vi "系统设置.vi"() -> ()   [LabVIEW 2016]
uses:
  <vilib>/Utility/miscctls.llb/LVPointTypeDef.ctl
  <vilib>/ptbypt/NI_PtbyPt.lvlib
  <vilib>/Utility/config.llb/NI_LVConfig.lvlib
  PLC/PLC.lvlib
panel:
  out "二级权限":bool
  in  "定时重启配置":bool
  in  "模块启用配置":bool
  in  "短信报警设置":bool
  in  "首页显示设置":bool
  in  "跨度核查":bool
  in  "空白核查":bool
  out "选项卡控件":enum32{"自由设定", "国标协议", "流量设定"}(tab)
  in  "24H周期设置":bool[](xcontrol)
  in  "运行间隔":i16=4 min=1 max=24
  in  "流量阈值":dbl=4.0 min=1.0 max=24.0
  in  "时间阈值":u16=4 min=1 max=24
  in  "周期设置":enum16{"自由设定", "国标协议", "流量设定"}(ring)
  out "一级权限":bool
  in  "质控启动日期":string(combo)="关闭"
  in  "跨度核查时间":u16(ring)=6 items=["00H", "01H", "02H", "03H", "04H", "05H", "06H", "07H", "08H", "09H", "10H", "11H", "12H", "13H", "14H", "15H", "16H", "17H", "18H", "19H", "20H", "21H", "22H", "23H", "关闭"]
  in  "空白核查时间":u16(ring)=2 items=["00H", "01H", "02H", "03H", "04H", "05H", "06H", "07H", "08H", "09H", "10H", "11H", "12H", "13H", "14H", "15H", "16H", "17H", "18H", "19H", "20H", "21H", "22H", "23H", "关闭"]
  in  "CODCr":bool
  in  "总磷总氮":bool
  in  "氨氮":bool
  in  "CODmn":bool
  in  "多参数":bool
  in  "输入密码":u32
  in  "布尔":bool
  in  "副屏显示设置":bool
  in  "开机启动":bool caption="氨氮禁用"
  in  "运行模式":enum16{"维护模式", "常规模式", "应急模式", "质控模式"}(ring)
  # "注：周期设置分为自由设定和国标协议两种。\n1：选择自由设定情况下：运行间隔将不可选用并变灰色，周期设置可自由手动勾选\n2：选择国标协议情况下：周期时间将由运行间隔选择的时间决定，下方周期设置被禁用并无法手动勾选。\n3：选择流量设定情况下：瞬时流量连续超过流量阈值到达时间阈值设定值，仪器将自动开启测量。"
  # "自动运行启动参数"
  # "质控频次："
  # "零点核查时间："
  # "跨度核查时间："
  # "启动周期设置"
  # "m3/S"
  # "秒"
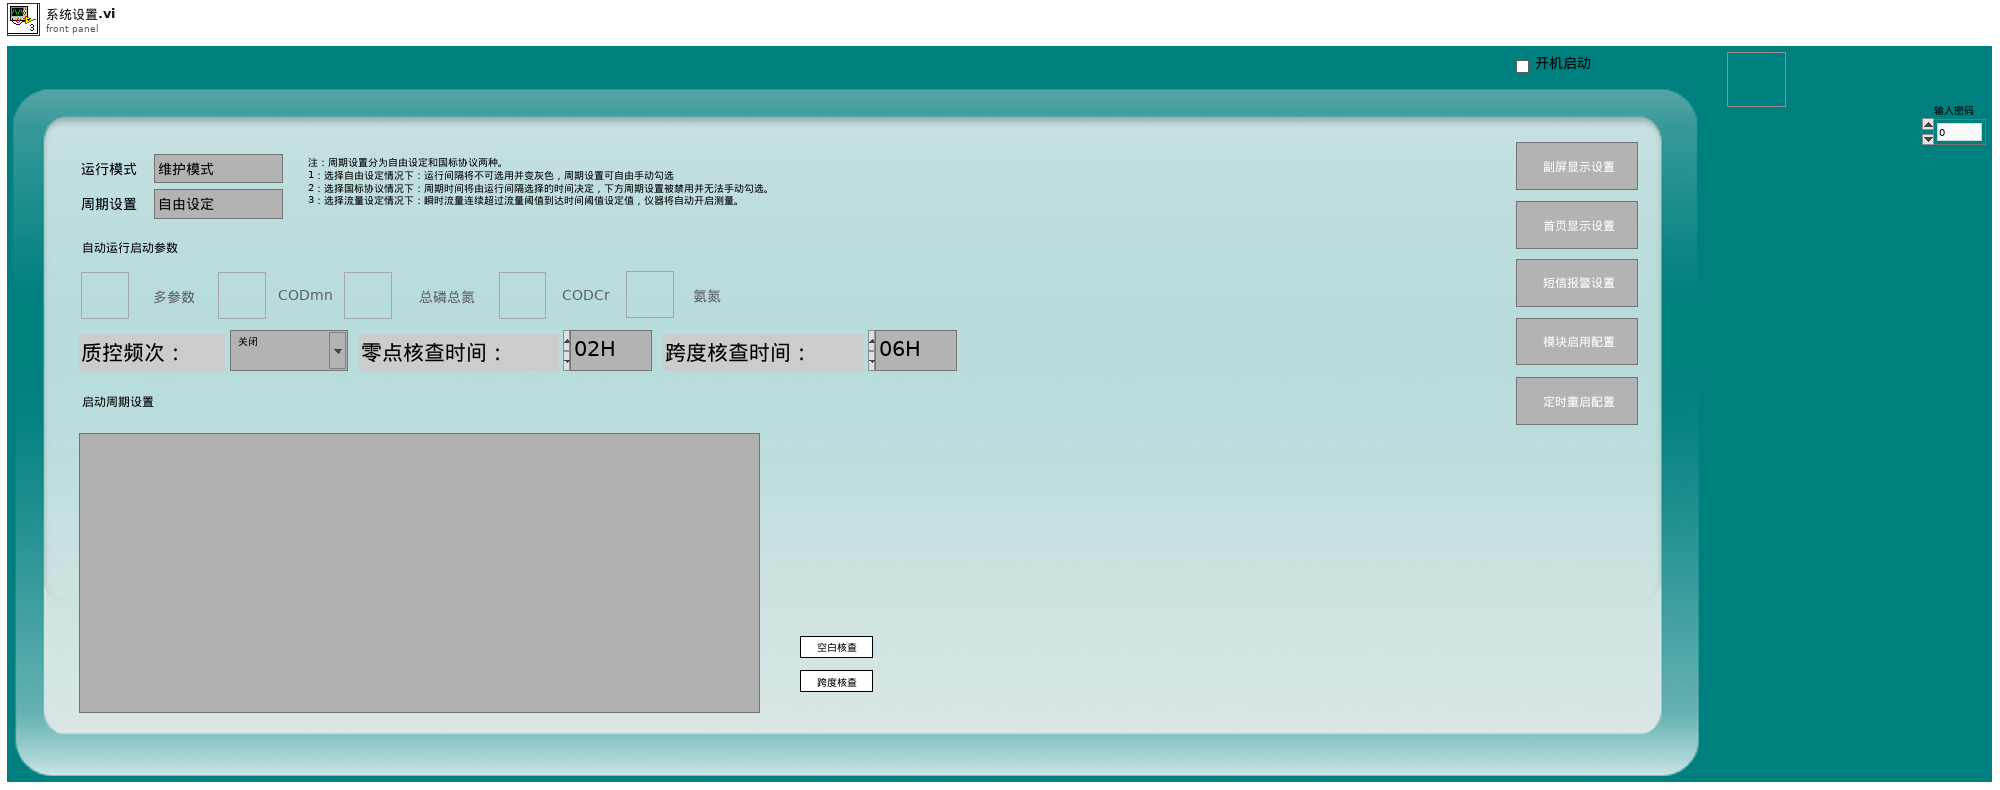
[diagram p1: front panel]
types:
  T1 = typedef "LVPointTypeDef.ctl" = cluster{"Horizontal":i16, "Vertical":i16}
  T2 = enum8{"Enabled", "Disabled", "Disabled and Grayed Out"}
  T3 = cluster{"频次":enum16{"关闭", "每天", "星期一", "星期二", "星期三", "星期四", "星期五", "星期六", "星期日"}, "时":u16, "分":u16}
  T4 = typedef "LVDateTimeRec.ctl" = cluster{"秒数的小数部分":dbl, "秒":i32, "分":i32, "时":i32, "日":i32, "月":i32, "年":i32, "天数（周）":i32, "天数（年）":i32, "DST":i32}
  T5 = enum16{"关闭", "每天", "星期一", "星期二", "星期三", "星期四", "星期五", "星期六", "星期日"}
  T6 = enum32{"Bad", "Idle", "Run top level", "Running"}
  T7 = typedef "NI_LVConfig.lvlib/Config Data RefNum.ctl" = refnum<k1>
  T8 = cluster{"运行模式":enum16{"维护模式", "常规模式", "应急模式", "质控模式"}}
  T9 = cluster{"测量模式":enum16{"水样测量", "标样核查", "零点核查", "跨度核查", "空白测试", "加标回收", "平行样", "校零", "校标"}}
  T10 = enum16{"启动测量", "标样核查", "零点核查", "跨度核查", "空白测试", "平行样测试", "加标回收", "空白校准", "标样校准", "初始化（清洗）", "停止测试", "仪器重启", "校时", "模式设置", "测量间隔设置"}
  T11 = cluster{"测试模式":enum16{"正常测试", "集成干预"}, "参数启用":cluster{"氨氮":bool, "总磷总氮":bool, "CODMn":bool, "CODcr":bool, "多参数":bool}}
  T12 = cluster{"运行模式":enum16{"维护模式", "常规模式", "应急模式", "质控模式"}, "质控频次":enum16{"关闭", "每天", "星期一", "星期二", "星期三", "星期四", "星期五", "星期六", "星期日"}, "空白核查时间":u16, "跨度核查时间":u16, "24H周期设置":bool[]}
  T13 = enum32{"Invalid", "Standard", "Closed", "Hidden", "Minimized", "Maximized"}
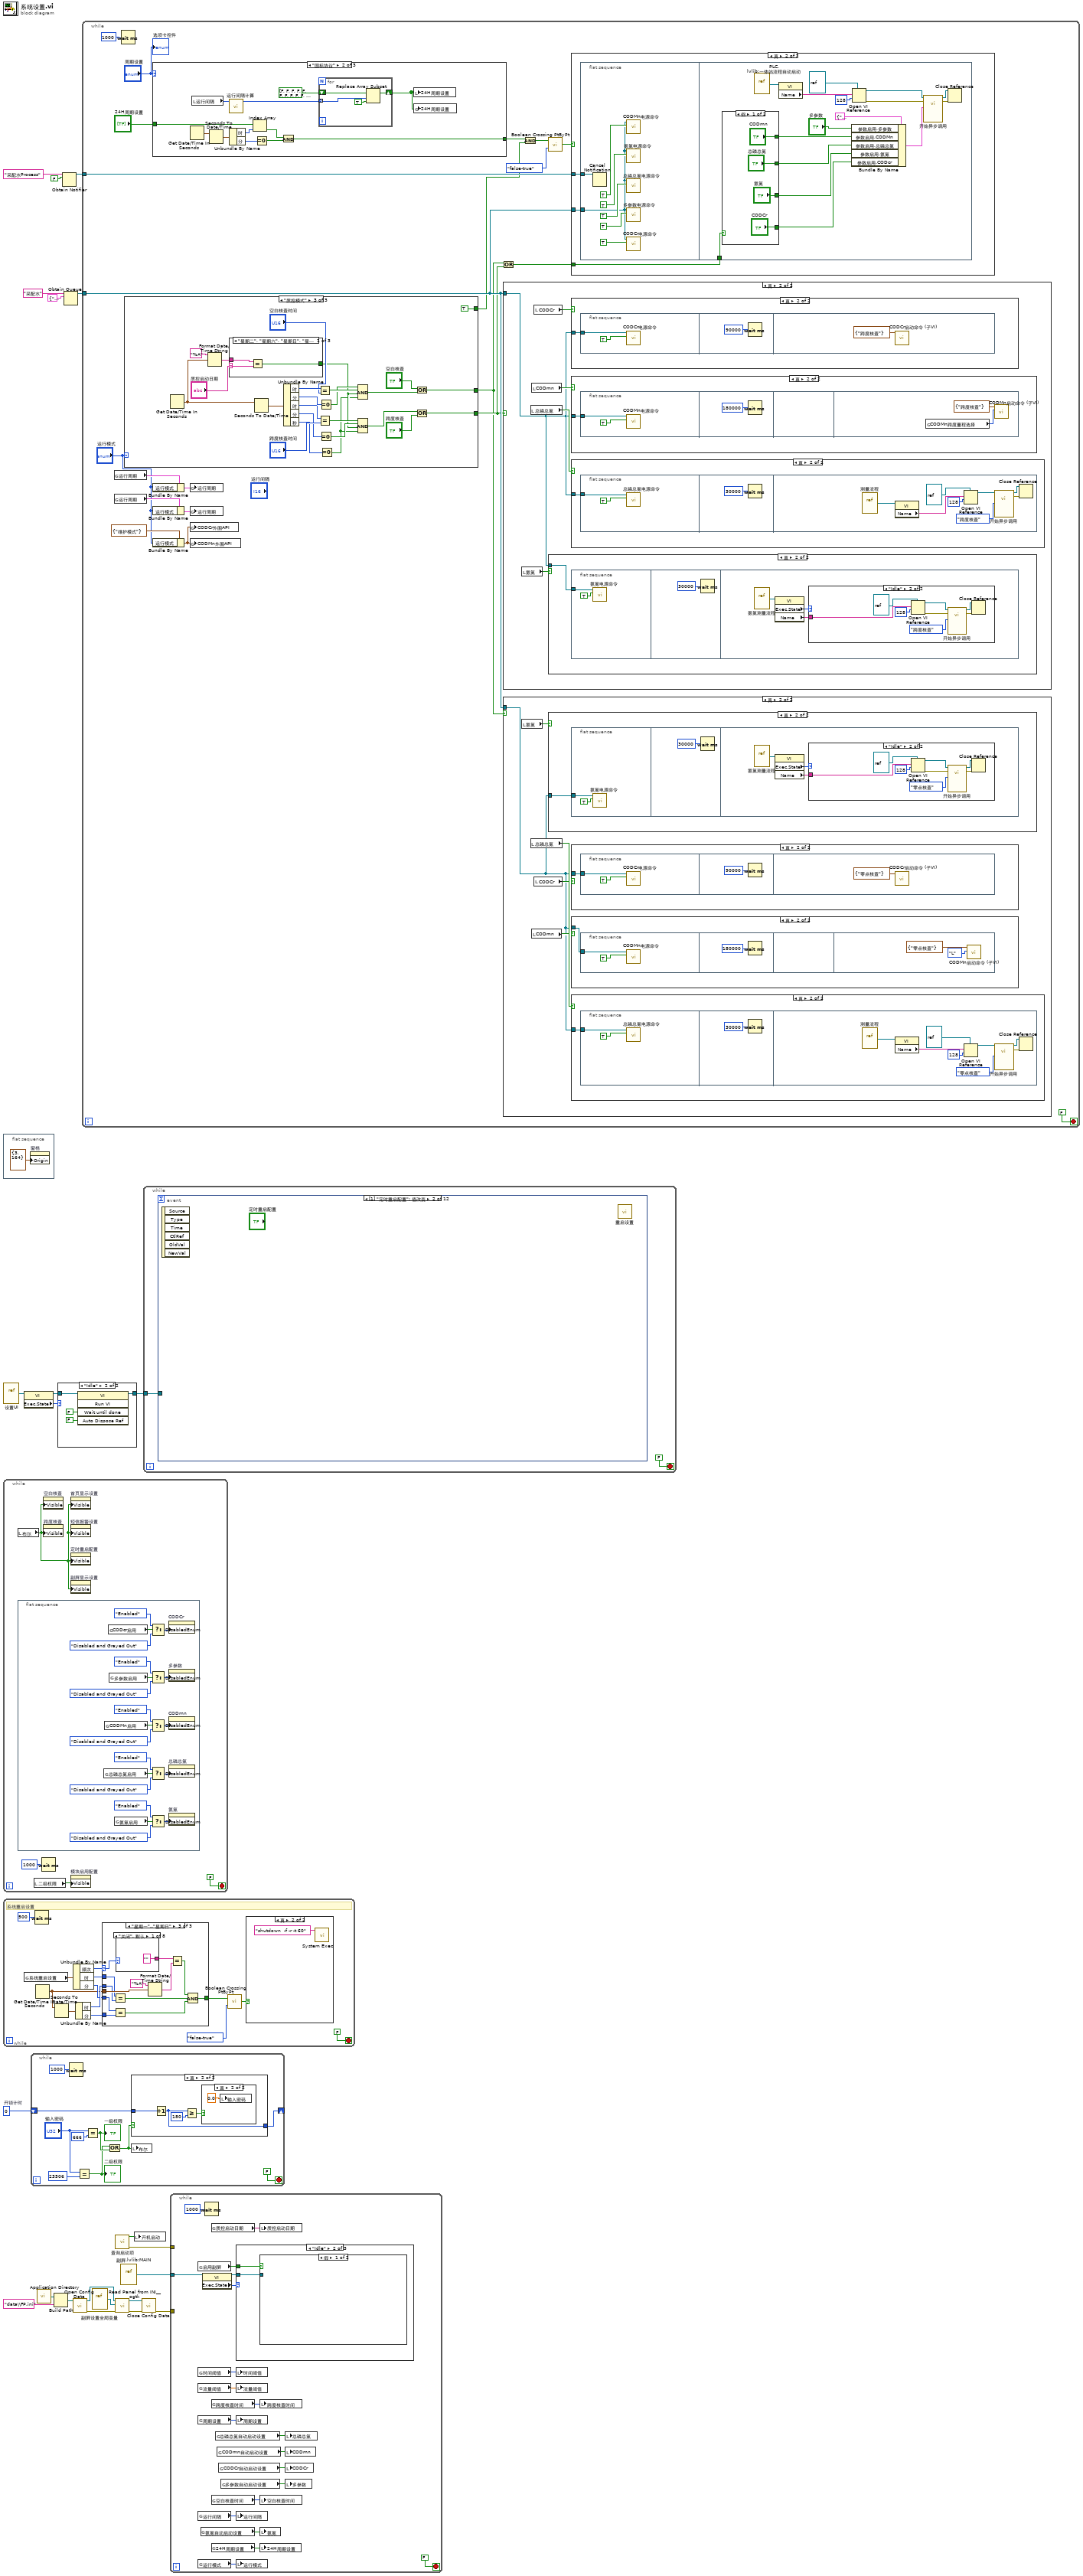
[diagram p0: block diagram]
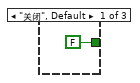
[diagram p3: hidden frame]
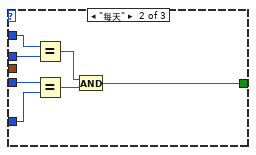
[diagram p4: hidden frame]
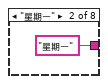
[diagram p5: hidden frame]
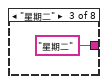
[diagram p6: hidden frame]
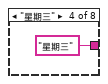
[diagram p7: hidden frame]
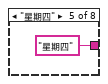
[diagram p8: hidden frame]
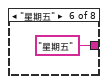
[diagram p9: hidden frame]
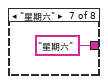
[diagram p10: hidden frame]
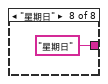
[diagram p11: hidden frame]
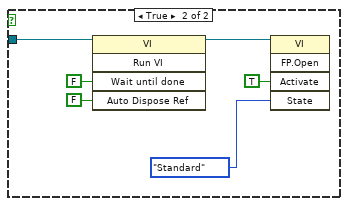
[diagram p16: hidden frame]
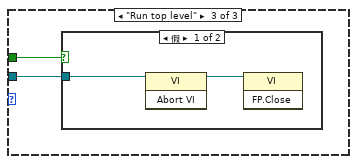
[diagram p17: hidden frame]
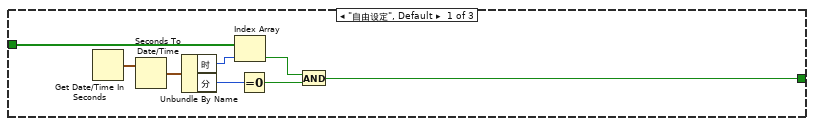
[diagram p19: hidden frame]
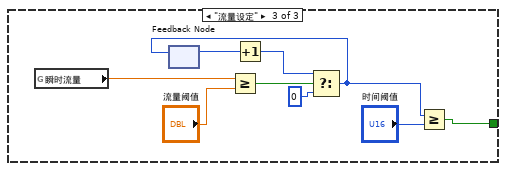
[diagram p20: hidden frame]
diagram:
  w19 = u32 0  # 开锁计时
  n1 = flat-sequence {
    frame #0 {
      n2 = property on="窗格" class="Pane"("Origin"=T1 {"Horizontal"=3, "Vertical"=164} ("原点")) -> ()  [unwired: 2 in, 2 out]
    }
  }
  n3 = vi-ref "设置UI.vi"() -> (w14:refnum<vi>)
  n4 = while {
    stop <- FALSE stop-if-true
    n5 = local read "布尔"() -> (w25:bool)
    n6 = flat-sequence {
      frame #0 {
        n7 = global read "系统设置全局变量.vi" "总磷总氮启用"() -> (w36:bool)
        n8 = global read "系统设置全局变量.vi" "CODMn启用"() -> (w34:bool)
        n9 = global read "系统设置全局变量.vi" "CODcr启用"() -> (w35:bool)
        n10 = global read "系统设置全局变量.vi" "多参数启用"() -> (w33:bool)
        n11 = global read "系统设置全局变量.vi" "氨氮启用"() -> (w29:bool)
        n12 = Select(t=T2."Enabled" ("禁用"), s=w35, f=T2."Disabled and Grayed Out" ("禁用")) -> (s? t:f=w48:T2)
        n13 = Select(t=T2."Enabled" ("禁用"), s=w33, f=T2."Disabled and Grayed Out" ("禁用")) -> (s? t:f=w32:T2)
        n14 = Select(t=T2."Enabled" ("禁用"), s=w34, f=T2."Disabled and Grayed Out" ("禁用")) -> (s? t:f=w38:T2)
        n15 = Select(t=T2."Enabled" ("禁用"), s=w36, f=T2."Disabled and Grayed Out" ("禁用")) -> (s? t:f=w31:T2)
        n16 = Select(t=T2."Enabled" ("禁用"), s=w29, f=T2."Disabled and Grayed Out" ("禁用")) -> (s? t:f=w37:T2)
        n17 = property on="CODCr" class="Bool (严格)"("DisabledEnum"=w48) -> ()  [unwired: 2 in, 2 out]
        n18 = property on="多参数" class="Bool (严格)"("DisabledEnum"=w32) -> ()  [unwired: 2 in, 2 out]
        n19 = property on="CODmn" class="Bool (严格)"("DisabledEnum"=w38) -> ()  [unwired: 2 in, 2 out]
        n20 = property on="总磷总氮" class="Bool (严格)"("DisabledEnum"=w31) -> ()  [unwired: 2 in, 2 out]
        n21 = property on="氨氮" class="Bool (严格)"("DisabledEnum"=w37) -> ()  [unwired: 2 in, 2 out]
      }
    }
    n22 = local read "二级权限"() -> (w26:bool)
    n23 = Wait (ms)(milliseconds to wait=u32 1000 ("等待时间（毫秒）")) -> ()  [unwired: 1 out]
    n24 = property on="空白核查" class="Bool"("Visible"=w25) -> ()  [unwired: 2 in, 2 out]
    n25 = property on="跨度核查" class="Bool"("Visible"=w25) -> ()  [unwired: 2 in, 2 out]
    n26 = property on="首页显示设置" class="Bool"("Visible"=w25) -> ()  [unwired: 2 in, 2 out]
    n27 = property on="短信报警设置" class="Bool"("Visible"=w25) -> ()  [unwired: 2 in, 2 out]
    n28 = property on="定时重启配置" class="Bool"("Visible"=w25) -> ()  [unwired: 2 in, 2 out]
    n29 = property on="副屏显示设置" class="Bool"("Visible"=w25) -> ()  [unwired: 2 in, 2 out]
    n30 = property on="模块启用配置" class="Bool"("Visible"=w26) -> ()  [unwired: 2 in, 2 out]
  }
  n31 = while {
    stop <- FALSE stop-if-true
    # "系统重启设置"
    n32 = global read "系统设置全局变量.vi" "系统重启设置"() -> (w61:T3)
    n33 = Wait (ms)(milliseconds to wait=u32 500 ("等待时间（毫秒）")) -> ()  [unwired: 1 out]
    n34 = Get Date/Time In Seconds() -> (seconds since 1Jan1904=w52:timestamp)
    n35 = Seconds To Date/Time(time stamp (now)=w52) -> (date time rec=w59:T4)  [unwired: 1 in]
    n36 = Unbundle By Name(w61) -> ("频次"=w60:T5, "时"=w56:u16, "分"=w55:u16)
    n37 = Unbundle By Name(w59) -> ("时"=w58:i32, "分"=w57:i32)
    n38 = case shown="\"星期一\"..\"星期日\"" w60 {
      selector: w60 -> [_ _ w81]
      tunnel: [FALSE w64 w71] -> w51
      tunnel: w58 -> [_ w70 w75]
      tunnel: w57 -> [_ w67 w73]
      tunnel: w56 -> [_ w69 w76]
      tunnel: w55 -> [_ w68 w74]
      tunnel: w52 -> [_ _ w82]
      frame "关闭", Default {
      }
      frame "每天" {
        n39 = Equal?(x=w69, y=w70) -> (x = y?=w65:bool)
        n40 = Equal?(x=w68, y=w67) -> (x = y?=w66:bool)
        n41 = And(x=w65, y=w66) -> (x .and. y?=w64:bool)
      }
      frame "星期一".."星期日" {
        n42 = Equal?(x=w76, y=w75) -> (x = y?=w77:bool)
        n43 = Equal?(x=w74, y=w73) -> (x = y?=w78:bool)
        n44 = case shown="\"关闭\", 默认" w81 {
          tunnel: ["" ("时间格式字符串(%c)") "星期一" ("时间格式字符串(%c)") "星期二" ("时间格式字符串(%c)") "星期三" ("时间格式字符串(%c)") "星期四" ("时间格式字符串(%c)") "星期五" ("时间格式字符串(%c)") "星期六" ("时间格式字符串(%c)") "星期日" ("时间格式字符串(%c)")] -> w79
          frame "关闭", Default {
          }
          frame "星期一" {
          }
          frame "星期二" {
          }
          frame "星期三" {
          }
          frame "星期四" {
          }
          frame "星期五" {
          }
          frame "星期六" {
          }
          frame "星期日" {
          }
        }
        n45 = Format Date/Time String(time format string (%c)="%A" ("时间格式字符串(%c)"), seconds (now)=w82) -> (date/time string=w80:string)  [unwired: 1 in]
        n46 = Equal?(x=w79, y=w80) -> (x = y?=w72:bool)
        n47 = Compound Arithmetic op=AND ("复合运算")(w72, w77, w78) -> (w71:bool)
      }
    }
    n48 = call <vilib>:"Boolean Crossing PtByPt.vi"("direction"=enum16{"either", "false-true", "true-false"}."false-true", "input"=w51) -> ("crossing"=w49:bool)  [unwired: 1 in]
    n49 = case shown="真" w49 {
      frame False {
      }
      frame True {
        n50 = call <vilib>:"System Exec.vi"("command line"="shutdown  -f -r -t 60") -> ()  [unwired: 7 in, 4 out]
      }
    }
  }
  n51 = property class="VI"(reference=w14) -> (reference out=w12:refnum<vi>, "Exec.State"=w13:T6)  [unwired: 1 in, 1 out]
  n52 = while {
    shift-right: [w97] -> _
    shift-left: w19 -> [w98]
    stop <- FALSE stop-if-true
    n53 = Wait (ms)(milliseconds to wait=u32 1000 ("等待时间（毫秒）")) -> ()  [unwired: 1 out]
    n54 = Equal?(x="输入密码", y=u32 23506) -> (x = y?=w92:bool)
    "二级权限" <- w92
    n55 = Equal?(x="输入密码", y=u32 666) -> (x = y?=w93:bool)
    "一级权限" <- w93
    n56 = Or(x=w92, y=w93) -> (x .or. y?=w94:bool)
    n57 = case shown="真" w94 {
      tunnel: w98 -> [_ w105]
      tunnel: [_ w104] -> w97
      frame False {
      }
      frame True {
        n58 = Increment(x=w105) -> (x+1=w104:u32)
        n59 = Greater Or Equal?(x=w104, y=u32 180) -> (x >= y?=w102:bool)
        n60 = case shown="真" w102 {
          frame False {
          }
          frame True {
            n61 = local write "输入密码"(0.0 ("输入密码")) -> ()
          }
        }
      }
    }
    n62 = local write "布尔"(w94) -> ()
  }
  n63 = call <vilib>:"Application Directory.vi"() -> ("Application Directory"=w1:path)
  n64 = Build Path(base path=w1, name or relative path="data\\FP.ini" ("名称或相对路径")) -> (appended path=w8:path)
  n65 = case shown="\"Idle\"" w13 {
    tunnel: w12 -> [w107 w111]
    tunnel: [w107 w110] -> w11
    frame "Bad", Default {
    }
    frame "Idle" {
      n66 = invoke class="VI" method="Run VI"(reference=w111, "Wait until done"=FALSE ("结束前等待"), "Auto Dispose Ref"=FALSE ("自动销毁引用")) -> (reference out=w110:refnum<vi>)  [unwired: 2 in, 4 out]
    }
  }
  n67 = Obtain Notifier(name (unnamed)="采配水Process" ("名称（未命名）"), notification data type=FALSE) -> (notifier out=w21:refnum<notifier>)  [unwired: 2 in, 2 out]
  n68 = Obtain Queue(name (unnamed)="采配水" ("名称（未命名）"), element data type=cluster{"命令":string, "数据":variant} {"命令"="", "数据"=variant}) -> (queue out=w16:refnum<queue>)  [unwired: 3 in, 2 out]
  n69 = call <vilib>:"Open Config Data.vi"("configuration file path"=w8) -> ("error out"=w7:errorcluster, "refnum"=w4:T7)  [unwired: 8 in, 1 out]
  n70 = while {
    tunnel: w21 -> [w130]
    tunnel: w16 -> [w126]
    stop <- FALSE stop-if-true
    n71 = global read "氨氮断电保存全局变量.vi" "运行周期"() -> (w116:T12)
    n72 = global read "总磷总氮断电保存全局变量.vi" "运行周期"() -> (w114:T12)
    n73 = Wait (ms)(milliseconds to wait=u32 1000 ("等待时间（毫秒）")) -> ()  [unwired: 1 out]
    n74 = case shown="\"质控模式\"" "运行模式" {
      tunnel: [_ _ w283] -> w119
      tunnel: [_ _ w287] -> w118
      tunnel: [_ TRUE TRUE] -> w123
      frame "维护模式", Default {
      }
      frame "常规模式" {
      }
      frame "质控模式" {
        n75 = Get Date/Time In Seconds() -> (seconds since 1Jan1904=w294:timestamp)
        n76 = Format Date/Time String(time format string (%c)="%A" ("时间格式字符串(%c)"), seconds (now)=w294) -> (date/time string=w292:string)  [unwired: 1 in]
        n77 = case shown="\"星期二\", \"星期六\", \"星期日\", \"星期三\", \"星期四\", \"星期五\", \"星期一\"" "质控启动日期" {
          selector: "质控启动日期" -> [w310 _ _]
          tunnel: [w309 TRUE FALSE] -> w295
          tunnel: w292 -> [w308 _ _]
          frame "星期二", "星期六", "星期日", "星期三", "星期四", "星期五", "星期一" {
            n78 = Equal?(x=w308, y=w310) -> (x = y?=w309:bool)
          }
          frame "每天" {
          }
          frame "关闭", Default {
          }
        }
        n79 = Seconds To Date/Time(time stamp (now)=w294) -> (date time rec=w307:T4)  [unwired: 1 in]
        n80 = Unbundle By Name(w307) -> ("时"=w306:i32, "分"=w304:i32, "时"=w300:i32, "分"=w299:i32, "秒"=w291:i32)
        n81 = Equal?(x=w306, y="空白核查时间") -> (x = y?=w303:bool)
        n82 = Equal?(x=w300, y="跨度核查时间") -> (x = y?=w298:bool)
        n83 = Equal To 0?(x=w304) -> (x = 0?=w302:bool)
        n84 = Equal To 0?(x=w299) -> (x = 0?=w297:bool)
        n85 = Equal To 0?(x=w291) -> (x = 0?=w290:bool)
        n86 = Compound Arithmetic op=AND ("复合运算")(w302, w303, w295, w290) -> (w288:bool)
        n87 = Compound Arithmetic op=AND ("复合运算")(w298, w297, w295, w290) -> (w285:bool)
        n88 = Or(x="空白核查", y=w288) -> (x .or. y?=w287:bool)
        n89 = Or(x=w285, y="跨度核查") -> (x .or. y?=w283:bool)
      }
    }
    n90 = case shown="\"国标协议\"" "周期设置" {
      tunnel: [w134 w141 w157] -> w122
      tunnel: "24H周期设置" -> [w133 w142 _]
      frame "自由设定", Default {
        n91 = Get Date/Time In Seconds() -> (seconds since 1Jan1904=w135:timestamp)
        n92 = Seconds To Date/Time(time stamp (now)=w135) -> (date time rec=w136:T4)  [unwired: 1 in]
        n93 = Unbundle By Name(w136) -> ("时"=w139:i32, "分"=w137:i32)
        n94 = Index Array(array=w133, index=w139) -> (element=w140:bool)
        n95 = Equal To 0?(x=w137) -> (x = 0?=w138:bool)
        n96 = And(x=w140, y=w138) -> (x .and. y?=w134:bool)
      }
      frame "国标协议" {
        n97 = Get Date/Time In Seconds() -> (seconds since 1Jan1904=w143:timestamp)
        n98 = local read "运行间隔"() -> (w152:i16)
        n99 = Seconds To Date/Time(time stamp (now)=w143) -> (date time rec=w144:T4)  [unwired: 1 in]
        n100 = call "运行间隔计算.vi"("运行周期"=w152) -> ("数组"=w151:i32[])  [unwired: 10 in]
        n101 = Unbundle By Name(w144) -> ("时"=w147:i32, "分"=w145:i32)
        n102 = Index Array(array=w142, index=w147) -> (element=w148:bool)
        n103 = Equal To 0?(x=w145) -> (x = 0?=w146:bool)
        n104 = And(x=w148, y=w146) -> (x .and. y?=w141:bool)
        n105 = for {
          tunnel: w151 -> [w155] mode=indexing
          shift-right: [w153] -> w149
          shift-left: bool[] [FALSE, FALSE, FALSE, FALSE, FALSE, FALSE, FALSE, FALSE, FALSE, FALSE, FALSE, FALSE, FALSE, FALSE, FALSE, FALSE, FALSE, FALSE, FALSE, FALSE, FALSE, FALSE, FALSE, FALSE] ("24H周期设置") -> [w156]
          n106 = Replace Array Subset(array=w156, new element=TRUE ("新元素/子数组"), index=w155) -> (w153:bool[])
        }
        n107 = local write "24H周期设置"(w149) -> ()
        n108 = global write "系统设置全局变量.vi" "24H周期设置"(w149) -> ()
      }
      frame "流量设定" {
        n109 = global read "流量计全局变量.vi" "瞬时流量"() -> (w165:dbl)
        n110 = feedback #1() -> (w162:i16)  [unwired: 1 in]
        n111 = Greater Or Equal?(x=w165, y="流量阈值") -> (x >= y?=w160:bool)
        n112 = Increment(x=w162) -> (x+1=w161:i16)
        n113 = Select(t=w161, s=w160, f=i16 0) -> (s? t:f=w159:i16)
        n114 = feedback-in #1(w159) -> ()
        n115 = Greater Or Equal?(x=w159, y="时间阈值") -> (x >= y?=w157:bool)
      }
    }
    n116 = Bundle By Name(cluster=w116, "运行模式"="运行模式") -> (w115:T12)
    n117 = Bundle By Name(cluster=w114, "运行模式"="运行模式") -> (w113:T12)
    n118 = Bundle By Name(cluster=T8 {"运行模式"=enum."维护模式"} ("外围API"), "运行模式"="运行模式") -> (w120:T8)
    n119 = global write "氨氮断电保存全局变量.vi" "运行周期"(w115) -> ()
    n120 = global write "总磷总氮断电保存全局变量.vi" "运行周期"(w113) -> ()
    n121 = global write "CODCr外部API.vi" "CODCr外围API"(w120) -> ()
    n122 = global write "CODMN外部API.vi" "CODMn外围API"(w120) -> ()
    n123 = Or(x=w118, y=w119) -> (x .or. y?=w117:bool)
    n124 = case shown="真" w119 {
      tunnel: w126 -> [_ w166]
      frame False {
      }
      frame True {
        n125 = local read "氨氮"() -> (w170:bool)
        n126 = local read "总磷总氮"() -> (w169:bool)
        n127 = local read "CODmn"() -> (w168:bool)
        n128 = local read "CODCr"() -> (w167:bool)
        n129 = case shown="真" w170 {
          tunnel: w166 -> [_ w194]
          frame False {
          }
          frame True {
            n130 = flat-sequence {
              tunnel: w194 -> [w195]
              frame #0 {
                n131 = call "氨氮电源命令.vi"("通电/断电"=TRUE, "队列"=w195) -> ()  [unwired: 9 in, 1 out]
              }
              frame #1 {
                n132 = Wait (ms)(milliseconds to wait=u32 30000 ("等待时间（毫秒）")) -> ()  [unwired: 1 out]
              }
              frame #2 {
                n133 = vi-ref "氨氮测量流程.vi"() -> (w200:refnum<vi>)
                n134 = property class="VI"(reference=w200) -> ("Exec.State"=w198:T6, "Name"=w199:string)  [unwired: 1 in, 2 out]
                n135 = case shown="\"Idle\"" w198 {
                  tunnel: w199 -> [_ w205]
                  frame "Bad", Default {
                  }
                  frame "Idle" {
                    n136 = Open VI Reference(type specifier VI Refnum (for type only)=refnum<vi> refnum, vi path=w205, options=128 ("选项")) -> (vi reference=w203:refnum<vi>, error out=w206:errorcluster)  [unwired: 3 in]
                    n137 = call-by-ref "开始异步调用"(reference=w203, error in=w206, "控制命令"=T10."跨度核查") -> (reference out=w207:refnum<vi>, error out=w208:errorcluster)  [unwired: 11 in]
                    n138 = Close Reference(reference=w207, error in (no error)=w208) -> ()  [unwired: 1 out]
                  }
                }
              }
            }
          }
        }
        n139 = case shown="真" w167 {
          tunnel: w166 -> [_ w171]
          frame False {
          }
          frame True {
            n140 = flat-sequence {
              tunnel: w171 -> [w172]
              frame #0 {
                n141 = call "CODCr电源命令.vi"("通电/断电"=TRUE, "队列"=w172) -> ()  [unwired: 9 in, 1 out]
              }
              frame #1 {
                n142 = Wait (ms)(milliseconds to wait=u32 90000 ("等待时间（毫秒）")) -> ()  [unwired: 1 out]
              }
              frame #2 {
                n143 = call "CODCr启动命令 (子VI).vi"("启动测量模式"=T9 {"测量模式"=enum."跨度核查"}) -> ()  [unwired: 11 in]
              }
            }
          }
        }
        n144 = case shown="真" w168 {
          tunnel: w166 -> [_ w176]
          frame False {
          }
          frame True {
            n145 = flat-sequence {
              tunnel: w176 -> [w177]
              frame #0 {
                n146 = call "CODMn电源命令.vi"("通电/断电"=TRUE, "队列"=w177) -> ()  [unwired: 9 in, 1 out]
              }
              frame #1 {
                n147 = Wait (ms)(milliseconds to wait=u32 180000 ("等待时间（毫秒）")) -> ()  [unwired: 1 out]
              }
              frame #2 {
              }
              frame #3 {
                n148 = global read "CODMn断电保存全局变量.vi" "CODMn跨度量程选择"() -> (w180:enum32{"H", "L", "AUTO"})
                n149 = call "CODMn启动命令 (子VI).vi"("CODMn量程切换"=w180, "启动测量模式"=T9 {"测量模式"=enum."跨度核查"}) -> ()  [unwired: 10 in]
              }
            }
          }
        }
        n150 = case shown="真" w169 {
          tunnel: w166 -> [_ w182]
          frame False {
          }
          frame True {
            n151 = flat-sequence {
              tunnel: w182 -> [w184]
              frame #0 {
                n152 = call "总磷总氮电源命令.vi"("通电/断电"=TRUE, "队列"=w184) -> ()  [unwired: 9 in, 1 out]
              }
              frame #1 {
                n153 = Wait (ms)(milliseconds to wait=u32 30000 ("等待时间（毫秒）")) -> ()  [unwired: 1 out]
              }
              frame #2 {
                n154 = vi-ref "测量流程.vi"() -> (w191:refnum<vi>)
                n155 = property class="VI"(reference=w191) -> ("Name"=w192:string)  [unwired: 1 in, 2 out]
                n156 = Open VI Reference(type specifier VI Refnum (for type only)=refnum<vi> refnum, vi path=w192, options=128 ("选项")) -> (vi reference=w190:refnum<vi>)  [unwired: 3 in, 1 out]
                n157 = call-by-ref "开始异步调用"(reference=w190, "控制命令"=T10."跨度核查") -> (reference out=w189:refnum<vi>, error out=w188:errorcluster)  [unwired: 12 in]
                n158 = Close Reference(reference=w189, error in (no error)=w188) -> ()  [unwired: 1 out]
              }
            }
          }
        }
      }
    }
    n159 = case shown="真" w118 {
      tunnel: w126 -> [_ w209]
      frame False {
      }
      frame True {
        n160 = local read "氨氮"() -> (w213:bool)
        n161 = local read "总磷总氮"() -> (w212:bool)
        n162 = local read "CODmn"() -> (w211:bool)
        n163 = local read "CODCr"() -> (w210:bool)
        n164 = case shown="真" w213 {
          tunnel: w209 -> [_ w237]
          frame False {
          }
          frame True {
            n165 = flat-sequence {
              tunnel: w237 -> [w238]
              frame #0 {
                n166 = call "氨氮电源命令.vi"("通电/断电"=TRUE, "队列"=w238) -> ()  [unwired: 9 in, 1 out]
              }
              frame #1 {
                n167 = Wait (ms)(milliseconds to wait=u32 30000 ("等待时间（毫秒）")) -> ()  [unwired: 1 out]
              }
              frame #2 {
                n168 = vi-ref "氨氮测量流程.vi"() -> (w243:refnum<vi>)
                n169 = property class="VI"(reference=w243) -> ("Exec.State"=w241:T6, "Name"=w242:string)  [unwired: 1 in, 2 out]
                n170 = case shown="\"Idle\"" w241 {
                  tunnel: w242 -> [_ w248]
                  frame "Bad", Default {
                  }
                  frame "Idle" {
                    n171 = Open VI Reference(type specifier VI Refnum (for type only)=refnum<vi> refnum, vi path=w248, options=128 ("选项")) -> (vi reference=w246:refnum<vi>, error out=w249:errorcluster)  [unwired: 3 in]
                    n172 = call-by-ref "开始异步调用"(reference=w246, error in=w249, "控制命令"=T10."零点核查") -> (reference out=w250:refnum<vi>, error out=w251:errorcluster)  [unwired: 11 in]
                    n173 = Close Reference(reference=w250, error in (no error)=w251) -> ()  [unwired: 1 out]
                  }
                }
              }
            }
          }
        }
        n174 = case shown="真" w210 {
          tunnel: w209 -> [_ w214]
          frame False {
          }
          frame True {
            n175 = flat-sequence {
              tunnel: w214 -> [w215]
              frame #0 {
                n176 = call "CODCr电源命令.vi"("通电/断电"=TRUE, "队列"=w215) -> ()  [unwired: 9 in, 1 out]
              }
              frame #1 {
                n177 = Wait (ms)(milliseconds to wait=u32 90000 ("等待时间（毫秒）")) -> ()  [unwired: 1 out]
              }
              frame #2 {
                n178 = call "CODCr启动命令 (子VI).vi"("启动测量模式"=T9 {"测量模式"=enum."零点核查"}) -> ()  [unwired: 11 in]
              }
            }
          }
        }
        n179 = case shown="真" w211 {
          tunnel: w209 -> [_ w219]
          frame False {
          }
          frame True {
            n180 = flat-sequence {
              tunnel: w219 -> [w220]
              frame #0 {
                n181 = call "CODMn电源命令.vi"("通电/断电"=TRUE, "队列"=w220) -> ()  [unwired: 9 in, 1 out]
              }
              frame #1 {
                n182 = Wait (ms)(milliseconds to wait=u32 180000 ("等待时间（毫秒）")) -> ()  [unwired: 1 out]
              }
              frame #2 {
              }
              frame #3 {
                n183 = call "CODMn启动命令 (子VI).vi"("CODMn量程切换"=enum32{"H", "L", "AUTO"}."L", "启动测量模式"=T9 {"测量模式"=enum."零点核查"}) -> ()  [unwired: 10 in]
              }
            }
          }
        }
        n184 = case shown="真" w212 {
          tunnel: w209 -> [_ w225]
          frame False {
          }
          frame True {
            n185 = flat-sequence {
              tunnel: w225 -> [w227]
              frame #0 {
                n186 = call "总磷总氮电源命令.vi"("通电/断电"=TRUE, "队列"=w227) -> ()  [unwired: 9 in, 1 out]
              }
              frame #1 {
                n187 = Wait (ms)(milliseconds to wait=u32 30000 ("等待时间（毫秒）")) -> ()  [unwired: 1 out]
              }
              frame #2 {
                n188 = vi-ref "测量流程.vi"() -> (w234:refnum<vi>)
                n189 = property class="VI"(reference=w234) -> ("Name"=w235:string)  [unwired: 1 in, 2 out]
                n190 = Open VI Reference(type specifier VI Refnum (for type only)=refnum<vi> refnum, vi path=w235, options=128 ("选项")) -> (vi reference=w233:refnum<vi>)  [unwired: 3 in, 1 out]
                n191 = call-by-ref "开始异步调用"(reference=w233, "控制命令"=T10."零点核查") -> (reference out=w232:refnum<vi>, error out=w231:errorcluster)  [unwired: 12 in]
                n192 = Close Reference(reference=w232, error in (no error)=w231) -> ()  [unwired: 1 out]
              }
            }
          }
        }
      }
    }
    n193 = And(x=w122, y=w123) -> (x .and. y?=w121:bool)
    n194 = call <vilib>:"Boolean Crossing PtByPt.vi"("direction"=enum16{"either", "false-true", "true-false"}."false-true", "input"=w121) -> ("crossing"=w128:bool)  [unwired: 1 in]
    n195 = case shown="真" w128 {
      tunnel: w130 -> [_ w254]
      tunnel: w126 -> [_ w253]
      tunnel: w117 -> [_ w252]
      frame False {
      }
      frame True {
        n196 = flat-sequence {
          tunnel: w254 -> [w261]
          tunnel: w253 -> [w255]
          tunnel: w252 -> [w262]
          frame #0 {
            n197 = Cancel Notification(0:w261) -> ()  [unwired: 1 in, 3 out]
            n198 = call "CODMn电源命令.vi"("通电/断电"=TRUE, "队列"=w255) -> ()  [unwired: 9 in, 1 out]
            n199 = call "氨氮电源命令.vi"("通电/断电"=TRUE, "队列"=w255) -> ()  [unwired: 9 in, 1 out]
            n200 = call "总磷总氮电源命令.vi"("通电/断电"=TRUE, "队列"=w255) -> ()  [unwired: 9 in, 1 out]
            n201 = call "多参数电源命令.vi"("通电/断电"=TRUE, "队列"=w255) -> ()  [unwired: 9 in, 1 out]
            n202 = call "CODCr电源命令.vi"("通电/断电"=TRUE, "队列"=w255) -> ()  [unwired: 9 in, 1 out]
          }
          frame #1 {
            n203 = case shown="假" w262 {
              tunnel: ["CODmn" _] -> w276
              tunnel: ["总磷总氮" _] -> w275
              tunnel: ["CODCr" _] -> w274
              tunnel: ["氨氮" _] -> w273
              frame False {
              }
              frame True {
              }
            }
            n204 = vi-ref "PLC.lvlib:一体站流程自动启动.vi"() -> (w270:refnum<vi>)
            n205 = property class="VI"(reference=w270) -> ("Name"=w271:string)  [unwired: 1 in, 2 out]
            n206 = Bundle By Name(cluster=T11 {"测试模式"=enum."正常测试", "参数启用"={"氨氮"=FALSE, "总磷总氮"=FALSE, "CODMn"=FALSE, "CODcr"=FALSE, "多参数"=FALSE}} ("参数"), "参数启用.多参数"="多参数", "参数启用.CODMn"=w276, "参数启用.总磷总氮"=w275, "参数启用.氨氮"=w273, "参数启用.CODcr"=w274) -> (w263:T11)
            n207 = Open VI Reference(type specifier VI Refnum (for type only)=refnum<vi> refnum, vi path=w271, options=128 ("选项")) -> (vi reference=w269:refnum<vi>, error out=w268:errorcluster)  [unwired: 3 in]
            n208 = call-by-ref "开始异步调用"(reference=w269, error in=w268, "参数"=w263) -> (reference out=w267:refnum<vi>, error out=w266:errorcluster)  [unwired: 11 in]
            n209 = Close Reference(reference=w267, error in (no error)=w266) -> ()  [unwired: 1 out]
          }
        }
      }
    }
    "选项卡控件" <- "周期设置"
  }
  n210 = vi-ref "副屏设置全局变量.vi"() -> (w5:refnum<vi>)
  n211 = call "查询启动项.vi"() -> ("error out"=w10:errorcluster, "包含启动项"=w20:bool)  [unwired: 10 in]
  n212 = call <userlib>:"Read Panel from INI__ogtk.vi"("error in (no error)"=w7, "VI ref"=w5, "refnum"=w4) -> ("error out"=w6:errorcluster, "refnum out"=w3:T7)  [unwired: 7 in]
  n213 = vi-ref "副屏.lvlib:MAIN.vi"() -> (w15:refnum<vi>)
  n214 = local write "开机启动"(w20) -> ()
  n215 = call <vilib>:"Close Config Data.vi"("error in (no error)"=w6, "refnum"=w3) -> ("error out"=w2:errorcluster)  [unwired: 8 in, 1 out]
  n216 = while {
    tunnel: w11 -> [w313]
    stop <- FALSE stop-if-true
    n217 = event shown="[1] \"定时重启配置\": 值改变" {
      selector: _ -> [_ _ _ _ _ _ _ _ _ _ _ _]
      dyn-events: _ -> [_ _ _ _ _ _ _ _ _ _ _ _]
      timeout: _ -> [_ _ _ _ _ _ _ _ _ _ _ _]
      tunnel: w313 -> [_ _ _ _ _ _ _ _ _ _ w367 _]
      event Timeout {
        n218 = event-data() -> ()  [unwired: 1 in, 3 out]
      }
      event "定时重启配置": Value Change {
        n219 = event-data() -> ()  [unwired: 1 in, 6 out]
        n220 = call "重启设置.vi"() -> ()  [unwired: 12 in]
      }
      event "模块启用配置": Value Change {
        n221 = event-data() -> ()  [unwired: 1 in, 6 out]
        n222 = call "模块启用配置框.vi"() -> ()  [unwired: 12 in]
      }
      event "24H周期设置", "运行模式", "多参数", "CODmn", "氨氮", "总磷总氮", "CODCr", "质控启动日期", "空白核查时间", "跨度核查时间", "运行间隔", "周期设置", "流量阈值", "时间阈值": Value Change {
        n223 = event-data() -> ()  [unwired: 1 in, 6 out]
        n224 = flat-sequence {
          frame #0 {
            n225 = local read "氨氮"() -> (w327:bool)
            n226 = local read "运行模式"() -> (w328:enum16{"维护模式", "常规模式", "应急模式", "质控模式"})
            n227 = local read "时间阈值"() -> (w316:u16)
            n228 = local read "周期设置"() -> (w317:enum16{"自由设定", "国标协议", "流量设定"})
            n229 = local read "总磷总氮"() -> (w325:bool)
            n230 = local read "流量阈值"() -> (w315:dbl)
            n231 = local read "运行间隔"() -> (w318:i16)
            n232 = local read "CODmn"() -> (w324:bool)
            n233 = local read "CODCr"() -> (w326:bool)
            n234 = local read "多参数"() -> (w323:bool)
            n235 = local read "跨度核查时间"() -> (w319:u16)
            n236 = local read "空白核查时间"() -> (w320:u16)
            n237 = local read "质控启动日期"() -> (w321:string)
            n238 = local read "24H周期设置"() -> (w322:bool[])
            n239 = global write "系统设置全局变量.vi" "氨氮自动启动设置"(w327) -> ()
            n240 = global write "系统设置全局变量.vi" "运行模式"(w328) -> ()
            n241 = global write "系统设置全局变量.vi" "多参数自动启动设置"(w323) -> ()
            n242 = global write "系统设置全局变量.vi" "时间阈值"(w316) -> ()
            n243 = global write "系统设置全局变量.vi" "CODmn自动启动设置"(w324) -> ()
            n244 = global write "系统设置全局变量.vi" "周期设置"(w317) -> ()
            n245 = global write "系统设置全局变量.vi" "总磷总氮自动启动设置"(w325) -> ()
            n246 = global write "系统设置全局变量.vi" "CODCr自动启动设置"(w326) -> ()
            n247 = global write "系统设置全局变量.vi" "流量阈值"(w315) -> ()
            n248 = global write "系统设置全局变量.vi" "运行间隔"(w318) -> ()
            n249 = global write "系统设置全局变量.vi" "跨度核查时间"(w319) -> ()
            n250 = global write "系统设置全局变量.vi" "空白核查时间"(w320) -> ()
            n251 = global write "系统设置全局变量.vi" "质控启动日期"(w321) -> ()
            n252 = global write "系统设置全局变量.vi" "24H周期设置"(w322) -> ()
          }
          frame #1 {
            n253 = call <vilib>:"Application Directory.vi"() -> ("Application Directory"=w342:path)
            n254 = Build Path(base path=w342, name or relative path="data\\sys.ini" ("名称或相对路径")) -> (appended path=w340:path)
            n255 = call <vilib>:"Open Config Data.vi"("configuration file path"=w340) -> ("error out"=w336:errorcluster, "refnum"=w339:T7)  [unwired: 8 in, 1 out]
            n256 = vi-ref "系统设置全局变量.vi"() -> (w338:refnum<vi>)
            n257 = call <userlib>:"Write Panel to INI__ogtk.vi"("error in (no error)"=w336, "VI ref"=w338, "refnum"=w339) -> ("error out"=w335:errorcluster, "refnum out"=w337:T7)  [unwired: 7 in]
            n258 = call <vilib>:"Close Config Data.vi"("error in (no error)"=w335, "refnum"=w337) -> ("error out"=w330:errorcluster, "file path"=w329:path)  [unwired: 8 in]
            n259 = Open/Create/Replace File(file path (use dialog)=w329, error in=w330) -> (refnum out=w333:refnum<file>, error out=w334:errorcluster)  [unwired: 4 in, 1 out]
            n260 = Flush File(refnum=w333, error in=w334) -> (refnum out=w332:refnum<file>, error out=w331:errorcluster)
            n261 = Close File(refnum=w332, error in=w331) -> ()  [unwired: 2 out]
          }
        }
      }
      event "运行间隔": Mouse Down {
        n262 = event-data() -> ("CtlRef"=w346:refnum<vi>)  [unwired: 1 in, 7 out]
        n263 = property class="DigNum (严格)"(reference=w346) -> (reference out=w345:refnum<vi>, "Value"=w344:i16)  [unwired: 1 in, 1 out]
        n264 = call "数字键盘.vi"("OldNumber"=w344) -> ("NewNumber"=w343:sgl)
        n265 = property class="DigNum (严格)"(reference=w345, "Val(Sgnl)"=w343) -> ()  [unwired: 1 in, 2 out]
      }
      event "流量阈值": Mouse Down {
        n266 = event-data() -> ("CtlRef"=w350:refnum<vi>)  [unwired: 1 in, 7 out]
        n267 = property class="DigNum (严格)"(reference=w350) -> (reference out=w349:refnum<vi>, "Value"=w348:dbl)  [unwired: 1 in, 1 out]
        n268 = call "数字键盘.vi"("OldNumber"=w348) -> ("NewNumber"=w347:sgl)
        n269 = property class="DigNum (严格)"(reference=w349, "Val(Sgnl)"=w347) -> ()  [unwired: 1 in, 2 out]
      }
      event "时间阈值": Mouse Down {
        n270 = event-data() -> ("CtlRef"=w354:refnum<vi>)  [unwired: 1 in, 7 out]
        n271 = property class="DigNum (严格)"(reference=w354) -> (reference out=w353:refnum<vi>, "Value"=w352:u16)  [unwired: 1 in, 1 out]
        n272 = call "数字键盘.vi"("OldNumber"=w352) -> ("NewNumber"=w351:sgl)
        n273 = property class="DigNum (严格)"(reference=w353, "Val(Sgnl)"=w351) -> ()  [unwired: 1 in, 2 out]
      }
      event "开机启动": Value Change {
        n274 = event-data() -> ("NewVal"=w356:bool)  [unwired: 1 in, 5 out]
        n275 = call <vilib>:"Application Directory.vi"() -> ("Application Directory"=w355:path)
        n276 = case shown="真" w356 {
          tunnel: w355 -> [w358 w362]
          frame False {
            n277 = call "删除启动项.vi"("启动文件路径"=w358) -> ("删除标记"=w357:bool)  [unwired: 9 in, 1 out]
            n278 = case shown="真" w357 {
              frame False {
                n279 = local write "开机启动"(TRUE ("开机启动")) -> ()
                n280 = One Button Dialog(message="启动项删除失败" ("消息")) -> ()  [unwired: 1 in, 1 out]
              }
              frame True {
              }
            }
          }
          frame True {
            n281 = call "添加启动项.vi"("启动文件路径"=w362) -> ("添加成功标记"=w361:bool)  [unwired: 9 in, 1 out]
            n282 = case shown="真" w361 {
              frame False {
                n283 = local write "开机启动"(FALSE ("开机启动")) -> ()
                n284 = One Button Dialog(message="启动项添加失败" ("消息")) -> ()  [unwired: 1 in, 1 out]
              }
              frame True {
              }
            }
          }
        }
      }
      event "副屏显示设置": Value Change {
        n285 = event-data() -> ()  [unwired: 1 in, 6 out]
        n286 = call "副屏设置.vi"() -> ()  [unwired: 12 in]
      }
      event "首页显示设置": Value Change {
        n287 = event-data() -> ()  [unwired: 1 in, 6 out]
        n288 = call "首页显示设置.vi"() -> ()  [unwired: 12 in]
      }
      event "短信报警设置": Value Change {
        n289 = event-data() -> ()  [unwired: 1 in, 6 out]
        n290 = invoke class="VI" method="FP.Open"(reference=w367, "Activate"=TRUE ("激活？"), "State"=T13."Standard" ("状态")) -> ()  [unwired: 2 in, 5 out]
      }
      event "布尔": Value Change {
        n291 = event-data() -> ("OldVal"=w369:bool)  [unwired: 1 in, 5 out]
        n292 = case shown="假" w369 {
          tunnel: [w370 _] -> w368
          frame False {
            n293 = call "数字密码键盘.vi"() -> ("NewNumber"=w370:sgl)  [unwired: 1 in]
          }
          frame True {
          }
        }
        n294 = local write "输入密码"(w368) -> ()
      }
    }
  }
  n295 = while {
    tunnel: w15 -> [w382]
    tunnel: w10 -> [_]
    tunnel: w2 -> [_]
    stop <- FALSE stop-if-true
    n296 = global read "副屏设置全局变量.vi" "启用副屏"() -> (w380:bool)
    n297 = global read "系统设置全局变量.vi" "时间阈值"() -> (w371:u16)
    n298 = global read "系统设置全局变量.vi" "流量阈值"() -> (w372:dbl)
    n299 = global read "系统设置全局变量.vi" "周期设置"() -> (w375:enum16{"自由设定", "国标协议", "流量设定"})
    n300 = global read "系统设置全局变量.vi" "运行间隔"() -> (w374:i16)
    n301 = global read "系统设置全局变量.vi" "运行模式"() -> (w373:enum16{"维护模式", "常规模式", "应急模式", "质控模式"})
    n302 = global read "系统设置全局变量.vi" "氨氮自动启动设置"() -> (w387:bool)
    n303 = property class="VI"(reference=w382) -> (reference out=w379:refnum<vi>, "Exec.State"=w381:T6)  [unwired: 1 in, 1 out]
    n304 = Wait (ms)(milliseconds to wait=u32 1000 ("等待时间（毫秒）")) -> ()  [unwired: 1 out]
    n305 = global read "系统设置全局变量.vi" "质控启动日期"() -> (w378:string)
    n306 = global read "系统设置全局变量.vi" "跨度核查时间"() -> (w376:u16)
    n307 = global read "系统设置全局变量.vi" "空白核查时间"() -> (w377:u16)
    n308 = global read "系统设置全局变量.vi" "24H周期设置"() -> (w388:bool[])
    n309 = global read "系统设置全局变量.vi" "总磷总氮自动启动设置"() -> (w385:bool)
    n310 = global read "系统设置全局变量.vi" "CODmn自动启动设置"() -> (w384:bool)
    n311 = global read "系统设置全局变量.vi" "CODCr自动启动设置"() -> (w386:bool)
    n312 = global read "系统设置全局变量.vi" "多参数自动启动设置"() -> (w383:bool)
    n313 = case shown="\"Idle\"" w381 {
      tunnel: w380 -> [_ w391 w399]
      tunnel: w379 -> [_ w392 w400]
      frame "Bad", Default {
      }
      frame "Idle" {
        n314 = case shown="假" w391 {
          tunnel: w392 -> [_ w398]
          frame False {
          }
          frame True {
            n315 = invoke class="VI" method="Run VI"(reference=w398, "Wait until done"=FALSE ("结束前等待"), "Auto Dispose Ref"=FALSE ("自动销毁引用")) -> (reference out=w393:refnum<vi>)  [unwired: 2 in, 4 out]
            n316 = invoke class="VI" method="FP.Open"(reference=w393, "Activate"=TRUE ("激活？"), "State"=T13."Standard" ("状态")) -> ()  [unwired: 2 in, 5 out]
          }
        }
      }
      frame "Run top level" {
        n317 = case shown="假" w399 {
          tunnel: w400 -> [w401 _]
          frame False {
            n318 = invoke class="VI" method="Abort VI"(reference=w401) -> (reference out=w402:refnum<vi>)  [unwired: 2 in, 2 out]
            n319 = invoke class="VI" method="FP.Close"(reference=w402) -> ()  [unwired: 2 in, 3 out]
          }
          frame True {
          }
        }
      }
    }
    n320 = local write "时间阈值"(w371) -> ()
    n321 = local write "流量阈值"(w372) -> ()
    n322 = local write "周期设置"(w375) -> ()
    n323 = local write "运行间隔"(w374) -> ()
    n324 = local write "运行模式"(w373) -> ()
    n325 = local write "质控启动日期"(w378) -> ()
    n326 = local write "跨度核查时间"(w376) -> ()
    n327 = local write "空白核查时间"(w377) -> ()
    n328 = local write "氨氮"(w387) -> ()
    n329 = local write "24H周期设置"(w388) -> ()
    n330 = local write "总磷总氮"(w385) -> ()
    n331 = local write "CODmn"(w384) -> ()
    n332 = local write "CODCr"(w386) -> ()
    n333 = local write "多参数"(w383) -> ()
  }
